vi "Jog_2Axis.vi"(0 "JOG_Up":bool, 1 "JOG_Down":bool, 2 "JOG_L":bool, 3 "JOG_R":bool, 4 "JOG_C+":bool, 5 "JOG_C-":bool, 6 "AxisArray":i32[](array[numeric]), 7 "Jog Ring":u16(ring) items=["Step", "Continuous"], 8 "ResolutionArray":dbl[](array[numeric]), 9 "Step Ring":u16(ring) items=["0.001 mm", "0.01 mm", "0.1 mm", "1 mm"], 11 "Jog_Speed":i32=10000) -> ()   [LabVIEW 2015]
uses:
  <userlib>/ADLINK/APS168.lvlib
panel:
  out "CurrentAxis":i32
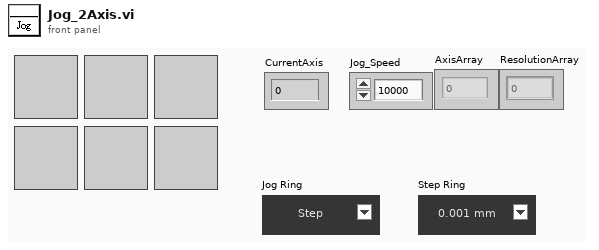
[diagram p1: front panel]
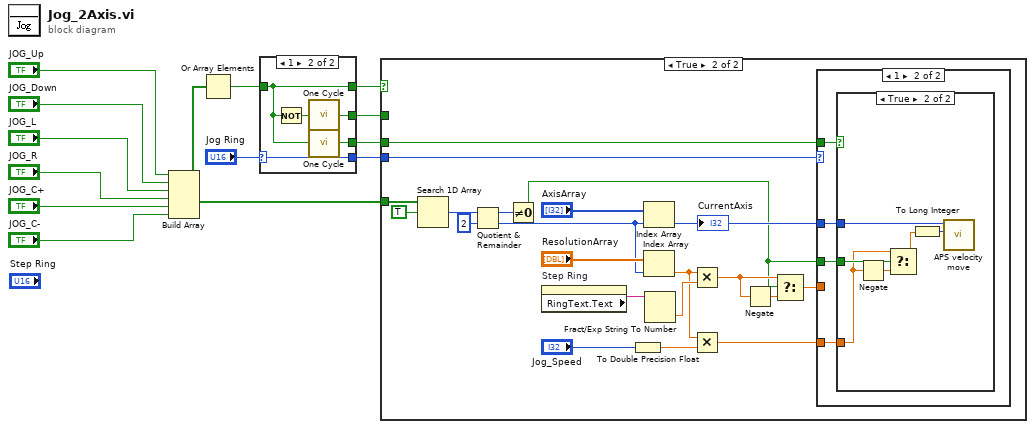
[diagram p0: block diagram]
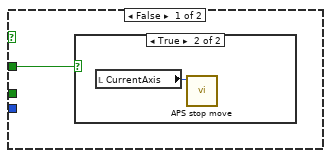
[diagram p2: hidden frame]
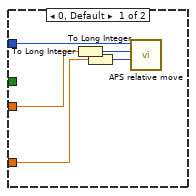
[diagram p4: hidden frame]
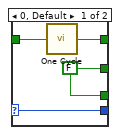
[diagram p6: hidden frame]
diagram:
  n1 = Build Array("JOG_Up", "JOG_Down", "JOG_L", "JOG_R", "JOG_C+", "JOG_C-") -> (w11:bool[])
  n2 = Or Array Elements(Boolean array=w11) -> (logical OR=w12:bool)
  n3 = case shown="1" "Jog Ring" {
    selector: "Jog Ring" -> [w14 w18]
    tunnel: w12 -> [w16 w21]
    tunnel: [w17 w21] -> w10
    tunnel: [w15 w20] -> w9
    tunnel: [w15 w19] -> w7
    tunnel: [w14 w18] -> w8
    frame 0, Default {
      w15 = FALSE ("Out")
      n4 = call "One Cycle.vi"("In"=w16) -> ("Out"=w17:bool)
    }
    frame 1 {
      n5 = Not(x=w21) -> (.not. x?=w22:bool)
      n6 = call "One Cycle.vi"("In"=w22) -> ("Out"=w20:bool)
      n7 = call "One Cycle.vi"("In"=w21) -> ("Out"=w19:bool)
    }
  }
  n8 = case shown="True" w10 {
    tunnel: w11 -> [_ w45]
    tunnel: w9 -> [w23 _]
    tunnel: w8 -> [_ w28]
    tunnel: w7 -> [_ w27]
    frame False {
      n9 = case shown="True" w23 {
        frame False {
        }
        frame True {
          n10 = local read "CurrentAxis"() -> (w24:i32)
          n11 = call <userlib>:"APS stop move.vi"("Axis_ID"=w24) -> ()  [unwired: 9 in, 2 out]
        }
      }
    }
    frame True {
      n12 = Search 1D Array(1D array=w45, element=TRUE) -> (index of element=w29:i32)  [unwired: 1 in]
      n13 = Quotient & Remainder(x=w29, y=2) -> (x-y*floor(x/y)=w38:i32, floor(x/y)=w25:i32)
      n14 = Not Equal To 0?(x=w38) -> (x != 0?=w26:bool)
      n15 = property on="Step Ring" class="Ring (strict)"() -> ("RingText.Text"=w37:string)  [unwired: 2 in, 2 out]
      n16 = To Double Precision Float(number="Jog_Speed") -> (double precision float=w30:dbl)
      n17 = Index Array(array="AxisArray", index=w25) -> (element=w40:i32)
      "CurrentAxis" <- w40
      n18 = Index Array(array="ResolutionArray", index=w25) -> (element=w33:dbl)
      n19 = Fract/Exp String To Number(string=w37) -> (number=w34:dbl)  [unwired: 3 in, 1 out]
      n20 = Multiply(x=w33, y=w34) -> (x*y=w35:dbl)
      n21 = Multiply(x=w33, y=w30) -> (x*y=w31:dbl)
      n22 = Negate(x=w35) -> (-x=w44:dbl)
      n23 = Select(t=w35, s=w26, f=w44) -> (s? t:f=w43:dbl)
      n24 = case shown="1" w28 {
        tunnel: w43 -> [w50 _]
        tunnel: w40 -> [w49 w53]
        tunnel: w31 -> [w48 w52]
        tunnel: w27 -> [_ w54]
        tunnel: w26 -> [_ w51]
        frame 0, Default {
          n25 = To Long Integer(number=w50) -> (32bit integer=w47:i32)
          n26 = To Long Integer(number=w48) -> (32bit integer=w46:i32)
          n27 = call <userlib>:"APS relative move.vi"("Max_Speed"=w46, "Distance"=w47, "Axis_ID"=w49) -> ()  [unwired: 7 in, 2 out]
        }
        frame 1 {
          n28 = case shown="True" w54 {
            tunnel: w53 -> [_ w60]
            tunnel: w52 -> [_ w57]
            tunnel: w51 -> [_ w58]
            frame False {
            }
            frame True {
              n29 = Negate(x=w57) -> (-x=w59:dbl)
              n30 = Select(t=w57, s=w58, f=w59) -> (s? t:f=w56:dbl)
              n31 = To Long Integer(number=w56) -> (32bit integer=w55:i32)
              n32 = call <userlib>:"APS velocity move.vi"("Max_Speed"=w55, "Axis_ID"=w60) -> ()  [unwired: 8 in, 2 out]
            }
          }
        }
      }
    }
  }
